vi "Close.vi"(8 "Error In":errorcluster, 11 "Draw Frame In":refnum<class "Draw Frame.lvclass">) -> (0 "Error Out":errorcluster)   [LabVIEW 2021, in "Draw Frame.lvclass"]
uses:
  Draw Frame.lvclass
  Process/Process.lvclass
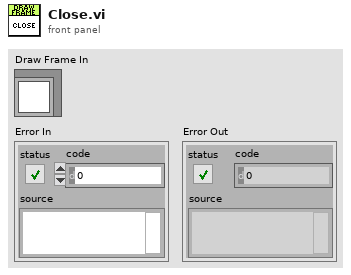
[diagram p1: front panel]
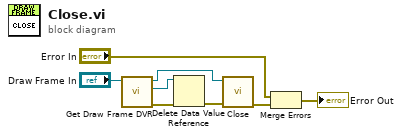
[diagram p0: block diagram]
diagram:
  n1 = call "Get Draw Frame DVR.vi"("Draw Frame In"="Draw Frame In") -> ("Error Out"=w4:errorcluster, "DVR"=w3:refnum<data-value>, "Draw Frame Out"=w1:refnum<class "Draw Frame.lvclass">)  [unwired: 8 in]
  n2 = Delete Data Value Reference(data value reference=w3, error in=w4) -> (error out=w2:errorcluster)  [unwired: 1 out]
  n3 = call-parent "Close.vi"("Error In"=w2, "Process In"=w1) -> ("Error Out"=w8:errorcluster)  [unwired: 9 in]
  n4 = Merge Errors("Error In", w8) -> (→"Error Out":errorcluster)
